vi "move_stage.vi"() -> ()   [LabVIEW 2014]
uses:
  C:/Program Files/Newport/Piezo Motion Control/Newport AG-UC2-UC8 Applet/Samples/LabVIEW 2009/AgilisCmdLib.dll
  Program Files/Newport/Piezo Motion Control/Newport AG-UC2-UC8 Applet/Samples/LabVIEW 2009/AgilisCmdLib.dll
panel:
  in  "Channel (1=cantilever, 2=dropper)":i32=1
  in  "Do Big step?":bool
  in  "Stop steps?":bool
  out "Doing step move?":bool
  in  "Delay Time (s)":dbl=1.0
  in  "Small step size":i64=-25
  in  "Max number of small steps":i32
  out "Doing initial move?":bool
  in  "Number of initial steps":i32=-24000
  out "ControllerVersion":string="AG-UC2 v2.2.0"
  out "VE":i32
  out "errstring 2":string
  out "PR":i32
  in  "Instrument Key":string="COM9"
  out "error out":errorcluster={"status"=TRUE, "code"=1172, "source"="Invoke Node Error calling method Newport.AgilisCmdLib.AgilisCmds.ML, (System.ArgumentNullException: Key cannot be null.\r\nParameter name: key) <append><b>System.ArgumentNullException</b> in move_stage.vi"}
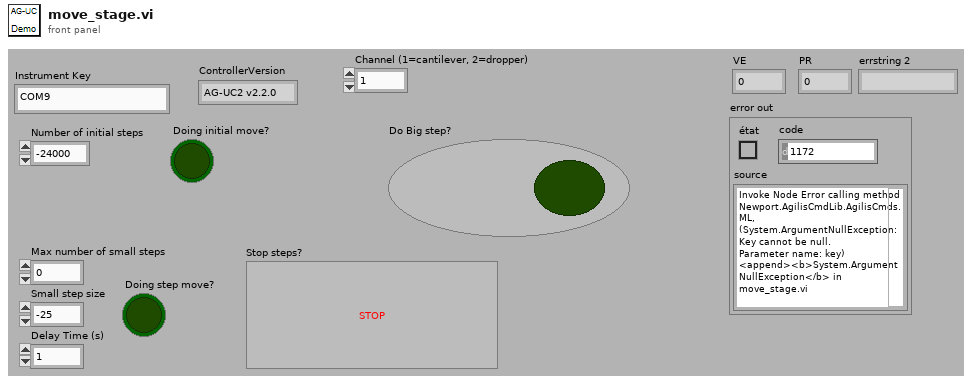
[diagram p1: front panel]
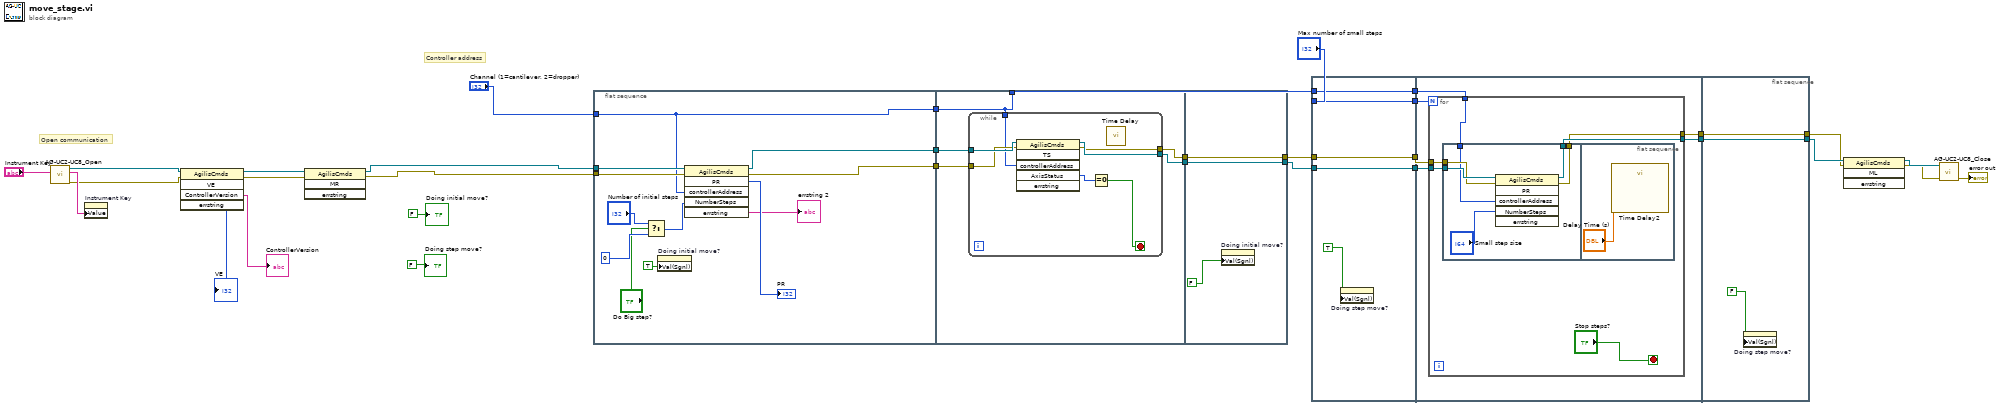
[diagram p0: block diagram]
diagram:
  # "Controller address"
  # "Open communication"
  n1 = call "AG-UC2-UC8_Open.vi"("Instrument Key IN"="Instrument Key") -> ("error out"=w30:errorcluster, "Instrument Key OUT"=w31:string, "AG-UC2-UC8 Reference"=w29:refnum<k24>)  [unwired: 3 in, 1 out]
  n2 = property on="Instrument Key" class="Str"("Value"=w31) -> ()  [unwired: 2 in, 2 out]
  n3 = invoke class="AgilisCmds" method="VE"(reference=w29, error in=w30) -> (reference out=w24:refnum<k24>, error out=w23:errorcluster, "VE"=→"VE":i32, "ControllerVersion"=→"ControllerVersion":string)  [unwired: 3 in, 1 out]
  n4 = invoke class="AgilisCmds" method="MR"(reference=w24, error in=w23) -> (reference out=w21:refnum<k24>, error out=w22:errorcluster)  [unwired: 2 in, 2 out]
  n5 = flat-sequence {
    tunnel: w22 -> [w43]
    tunnel: w21 -> [w42]
    tunnel: "Channel (1=cantilever, 2=dropper)" -> [w41]
    tunnel: [w41] -> w19
    tunnel: [w40] -> w18
    tunnel: [w39] -> w17
    tunnel: w19 -> [w46]
    tunnel: w18 -> [w48]
    tunnel: w17 -> [w47]
    tunnel: [w50] -> w16
    tunnel: [w49] -> w15
    tunnel: [w46] -> w11
    tunnel: [w59] -> w12
    tunnel: [w60] -> w13
    tunnel: w16 -> [w60]
    tunnel: w15 -> [w59]
    frame #0 {
      n6 = Select(t="Number of initial steps", s="Do Big step?", f=0) -> (s? t:f=w37:i32)
      n7 = property on="Doing initial move?" class="Bool (strict)"("Val(Sgnl)"=TRUE ("Value (Signaling)")) -> ()  [unwired: 2 in, 2 out]
      n8 = invoke class="AgilisCmds" method="PR"(reference=w42, error in=w43, "controllerAddress"=w41, "NumberSteps"=w37) -> (reference out=w40:refnum<k24>, error out=w39:errorcluster, "PR"=→"PR":i32, "errstring"=→"errstring 2":string)  [unwired: 2 in, 2 out]
    }
    frame #1 {
      n9 = while {
        tunnel: w48 -> [w57]
        tunnel: w47 -> [w56]
        tunnel: w46 -> [w55]
        tunnel: [w52] -> w50
        tunnel: [w51] -> w49
        stop <- w53 stop-if-true
        n10 = invoke class="AgilisCmds" method="TS"(reference=w57, error in=w56, "controllerAddress"=w55) -> (reference out=w52:refnum<k24>, error out=w51:errorcluster, "AxisStatus"=w54:i32)  [unwired: 3 in, 3 out]
        n11 = Equal To 0?(x=w54) -> (x = 0?=w53:bool)
        n12 = call "Time Delay"() -> ()  [unwired: 11 in, 1 out]
      }
    }
    frame #2 {
      n13 = property on="Doing initial move?" class="Bool (strict)"("Val(Sgnl)"=FALSE ("Value (Signaling)")) -> ()  [unwired: 2 in, 2 out]
    }
  }
  n14 = flat-sequence {
    tunnel: w11 -> [w62]
    tunnel: w12 -> [w63]
    tunnel: w13 -> [w64]
    tunnel: "Max number of small steps" -> [w65]
    tunnel: [w65] -> w8
    tunnel: [w64] -> w7
    tunnel: [w63] -> w6
    tunnel: [w62] -> w5
    tunnel: w8 -> [w71]
    tunnel: w7 -> [w70]
    tunnel: w6 -> [w69]
    tunnel: w5 -> [w68]
    tunnel: [w67] -> w4
    tunnel: [w66] -> w3
    tunnel: [w86] -> w9
    tunnel: [w87] -> w10
    tunnel: w4 -> [w87]
    tunnel: w3 -> [w86]
    frame #0 {
      n15 = property on="Doing step move?" class="Bool (strict)"("Val(Sgnl)"=TRUE ("Value (Signaling)")) -> ()  [unwired: 2 in, 2 out]
    }
    frame #1 {
      n16 = for {
        N: w71 -> [_]
        tunnel: w70 -> [w77]
        tunnel: w69 -> [w76]
        tunnel: w68 -> [w75]
        tunnel: [w74] -> w67
        tunnel: [w73] -> w66
        stop <- "Stop steps?" stop-if-true
        n17 = flat-sequence {
          tunnel: w77 -> [w83]
          tunnel: w76 -> [w82]
          tunnel: w75 -> [w81]
          tunnel: [w79] -> w74
          tunnel: [w78] -> w73
          frame #0 {
            n18 = invoke class="AgilisCmds" method="PR"(reference=w83, error in=w82, "controllerAddress"=w81, "NumberSteps"="Small step size") -> (reference out=w79:refnum<k24>, error out=w78:errorcluster)  [unwired: 2 in, 4 out]
          }
          frame #1 {
            n19 = call "Time Delay2"("Delay Time (s)"="Delay Time (s)") -> ()  [unwired: 10 in, 1 out]
          }
        }
      }
    }
    frame #2 {
      n20 = property on="Doing step move?" class="Bool (strict)"("Val(Sgnl)"=FALSE ("Value (Signaling)")) -> ()  [unwired: 2 in, 2 out]
    }
  }
  n21 = invoke class="AgilisCmds" method="ML"(reference=w10, error in=w9) -> (reference out=w26:refnum<k24>, error out=w25:errorcluster)  [unwired: 2 in, 2 out]
  n22 = call "AG-UC2-UC8_Close.vi"("error in (no error)"=w25, "AG-UC2-UC8 Reference"=w26) -> ("Error out"=→"error out":errorcluster)  [unwired: 2 in, 1 out]
  "Doing initial move?" <- FALSE ("Boolean")
  "Doing step move?" <- FALSE ("Boolean")
